vi "INSERT INTO DB.vi"(8 "error in":errorcluster, 10 "object":refnum<class "_ISerializable.lvclass">, 11 "orm in":refnum<class "LV-ORM.lvclass">) -> (0 "error out":errorcluster, 3 "orm out":refnum<class "LV-ORM.lvclass">)   [LabVIEW 2018, in "LV-ORM.lvclass"]
uses:
  LV-ORM.lvclass
  _Serializable Base Object/_ISerializable.lvclass
  <vilib>/NI/Configuration Framework/class discovery singleton/class discovery singleton.lvlib
  Serializer/Serializer.lvclass
panel:
  out "INSERT script":string
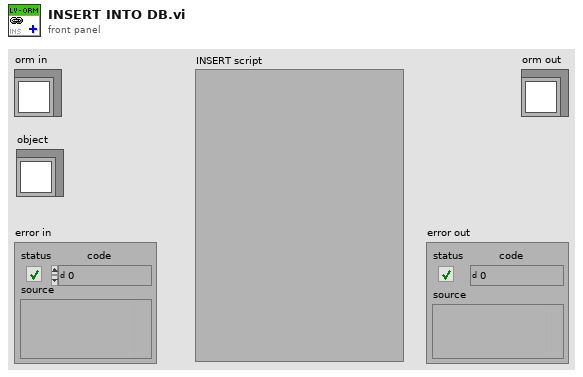
[diagram p1: front panel]
types:
  T1 = typedef "key-value-type cluster.ctl" = cluster{"names":string[], "values":string[], "type":string[], "class name":string}
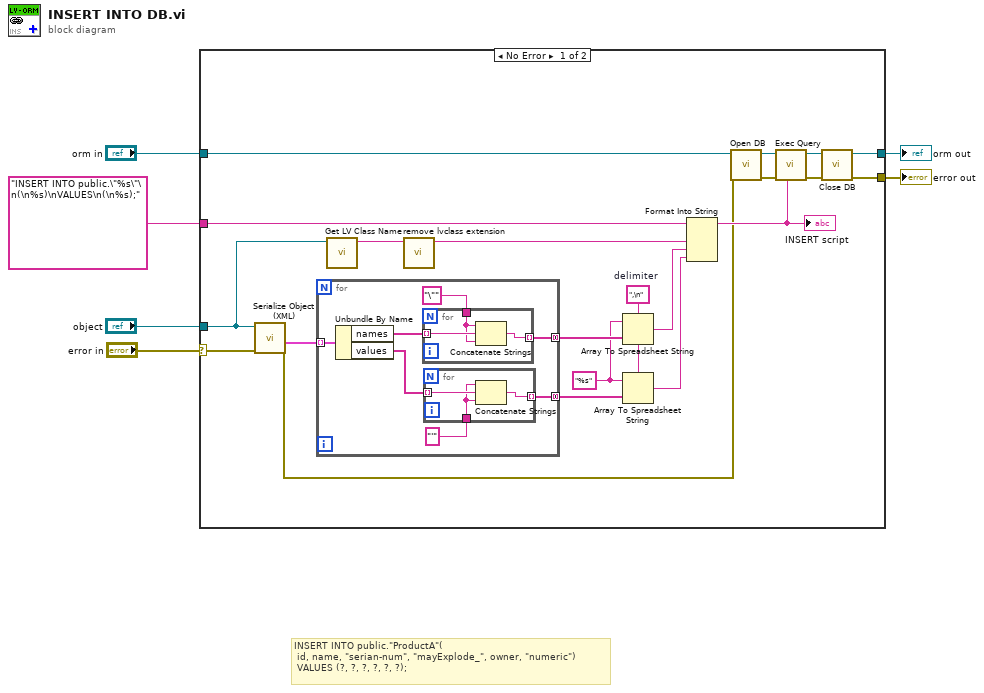
[diagram p0: block diagram]
diagram:
  # "INSERT INTO public.\"ProductA\"(\n\tid, name, \"serian-num\", \"mayExplode_\", owner, \"numeric\")\n\tVALUES (?, ?, ?, ?, ?, ?);"
  n1 = case shown="No Error" "error in" {
    selector: "error in" -> [w7 w42]
    tunnel: "INSERT INTO public.\"%s\"\n(\n%s)\nVALUES\n(\n%s);" -> [w27 _]
    tunnel: "orm in" -> [w23 w41]
    tunnel: [w22 w41] -> w4
    tunnel: [w21 w42] -> w3
    tunnel: "object" -> [w20 _]
    frame No Error {
      w13 = "%s"
      w18 = ",\n"  # delimiter
      n2 = call "Serialize Object (XML).vi"("error in"=w7, "object in"=w20) -> ("error out"=w12:errorcluster, "key-value-type"=w24:T1[])  [unwired: 5 in, 3 out]
      n3 = for {
        tunnel: w24 -> [w34] mode=indexing
        tunnel: [w33] -> w19 mode=concatenating
        tunnel: [w32] -> w14 mode=concatenating
        n4 = Unbundle By Name(w34) -> ("names"=w31:string[], "values"=w30:string[])
        n5 = for {
          tunnel: w31 -> [w40] mode=indexing
          tunnel: [w39] -> w33 mode=indexing
          tunnel: "\"" -> [w38]
          n6 = Concatenate Strings(w38, w40, w38) -> (w39:string)
        }
        n7 = for {
          tunnel: w30 -> [w37] mode=indexing
          tunnel: [w36] -> w32 mode=indexing
          tunnel: "'" -> [w35]
          n8 = Concatenate Strings(w35, w37, w35) -> (w36:string)
        }
      }
      n9 = call <vilib>:"Get LV Class Name.vi"("object"=w20) -> ("class name"=w26:string)  [unwired: 9 in, 1 out]
      n10 = call <vilib>:"remove lvclass extension.vi"("class name in"=w26) -> ("class name out"=w25:string)  [unwired: 10 in]
      n11 = Array To Spreadsheet String(delimiter (Tab)=w18, array=w19, 3:w13) -> (spreadsheet string=w17:string)
      n12 = Array To Spreadsheet String(delimiter (Tab)=w18, array=w14, 3:w13) -> (spreadsheet string=w16:string)
      n13 = Format Into String(format string=w27, w25, w17, w16) -> (resulting string=w15:string)  [unwired: 2 in, 1 out]
      "INSERT script" <- w15
      n14 = call "Open DB.vi"("error in (no error)"=w12, "LV-ORM in"=w23) -> ("error out"=w8:errorcluster, "LV-ORM out"=w11:refnum<class "LV-ORM.lvclass">)  [unwired: 8 in]
      n15 = call "Exec Query.vi"("scripts"=w15, "error in"=w8, "orm in"=w11) -> ("error out"=w9:errorcluster, "orm out"=w10:refnum<class "LV-ORM.lvclass">)  [unwired: 7 in]
      n16 = call "Close DB.vi"("error in"=w9, "LV-ORM in"=w10) -> ("error out"=w21:errorcluster, "LV-ORM out"=w22:refnum<class "LV-ORM.lvclass">)  [unwired: 8 in]
    }
    frame Error {
    }
  }
  "orm out" <- w4
  "error out" <- w3
